vi "u32-u8s.vi"(10 "数值":u32) -> (2 "反转的数组":u8[](array[numeric]))   [LabVIEW 2012]
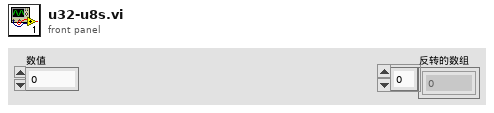
[diagram p1: front panel]
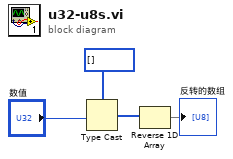
[diagram p0: block diagram]
diagram:
  n1 = Type Cast(type=u8[] [], x="数值") -> (*(type *) &x=w2:u8[])
  n2 = Reverse 1D Array(array=w2) -> (reversed array=→"反转的数组":u8[])
